vi "TCP_DATA_Subscriber_subVi_copy2.vi"(8 "error in":errorcluster, 10 "data String":refnum<vi>, 11 "connection ID":refnum<k5>) -> (0 "error out":errorcluster={"status"=TRUE, "code"=66, "source"="TCP Read in test_DATA_TCP_client.vi"})   [LabVIEW 2013]
panel:
  out "after substring":string
  out "array":dbl[](graph)
  out "time string":string="4:31 PM"
  out "data out":string
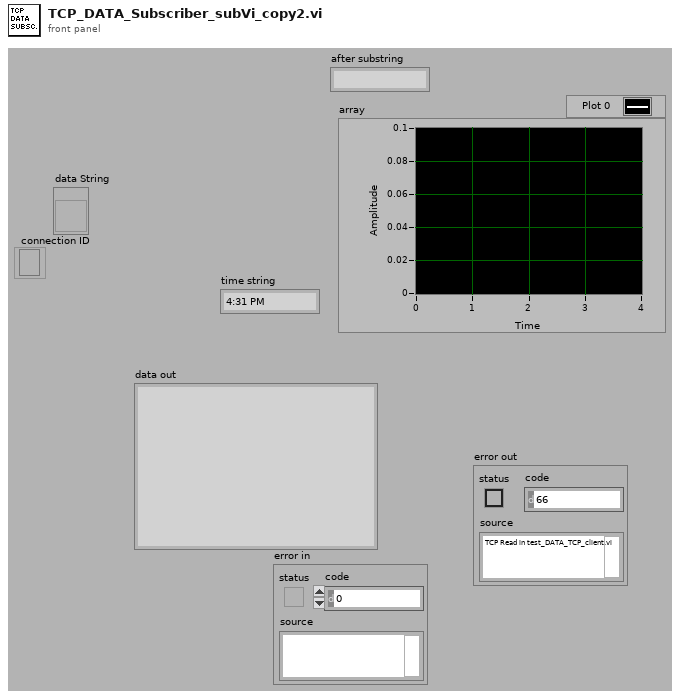
[diagram p1: front panel]
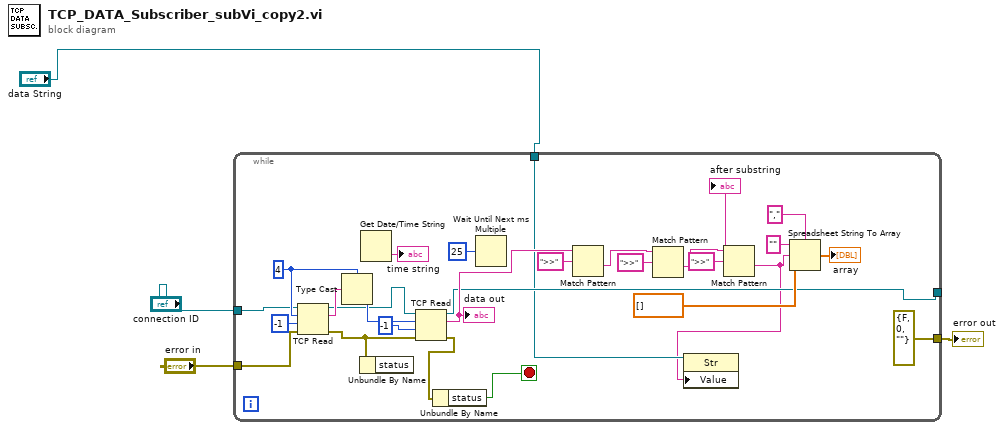
[diagram p0: block diagram]
diagram:
  n1 = while {
    tunnel: "error in" -> [w25]
    tunnel: "connection ID" -> [w23]
    tunnel: [errorcluster {"status"=FALSE, "code"=0, "source"=""} ("error out")] -> w1
    tunnel: [w10] -> _
    tunnel: "data String" -> [w9]
    stop <- w6 stop-if-true
    w30 = 4
    n2 = TCP Read(connection ID=w23, bytes to read=w30, error in (no error)=w25, 9:-1 ("timeout ms (25000)")) -> (connection ID out=w27:refnum<k5>, data out=w29:string, error out=w24:errorcluster)  [unwired: 1 in]
    n3 = Type Cast(type=w30, x=w29) -> (*(type *) &x=w28:i32)
    n4 = Unbundle By Name(w24) -> ()  [unwired: 1 out]
    n5 = Get Date/Time String() -> (time string=→"time string":string)  [unwired: 3 in, 1 out]
    n6 = TCP Read(connection ID=w27, bytes to read=w28, error in (no error)=w24, 9:-1) -> (connection ID out=w10:refnum<k5>, data out=w20:string, error out=w7:errorcluster)  [unwired: 1 out]
    "data out" <- w20
    n7 = Unbundle By Name(w7) -> ("status"=w6:bool)
    n8 = Wait Until Next ms Multiple(millisecond multiple=u32 25) -> ()  [unwired: 1 out]
    n9 = Match Pattern(string=w20, regular expression=">>") -> (after substring=w17:string)  [unwired: 1 in, 3 out]
    n10 = Match Pattern(string=w17, regular expression=">>") -> (after substring=w15:string)  [unwired: 1 in, 3 out]
    n11 = Match Pattern(string=w15, regular expression=">>") -> (after substring=w8:string)  [unwired: 1 in, 3 out]
    "after substring" <- w8
    n12 = property class="Str"(reference=w9, "Value"=w8) -> ()  [unwired: 1 in, 2 out]
    n13 = Spreadsheet String To Array(delimiter (Tab)=",", format string="", spreadsheet string=w8, array type (2D Dbl)=dbl[] []) -> (array=→"array":dbl[])
  }
  "error out" <- w1
